vi "Parse Response Message.vi"(6 "Command in":T1, 8 "error in":errorcluster, 11 "Kronos in":refnum<class "Kronos.lvclass">) -> (0 "error out":errorcluster, 3 "Kronos out":refnum<class "Kronos.lvclass">)   [LabVIEW 2018, in "Kronos.lvlib" / "Kronos.lvclass"]
uses:
  Kronos.lvclass
  PPLs/Laser/Parent/Laser.lvlibp/Custom Controls/Command List.ctl
  PPLs/Laser/Parent/Laser.lvlibp/Laser.lvclass
  C:/AME Test Engineering/LabVIEW/PPLs/Laser/Parent/Laser.lvlibp/Laser.lvclass
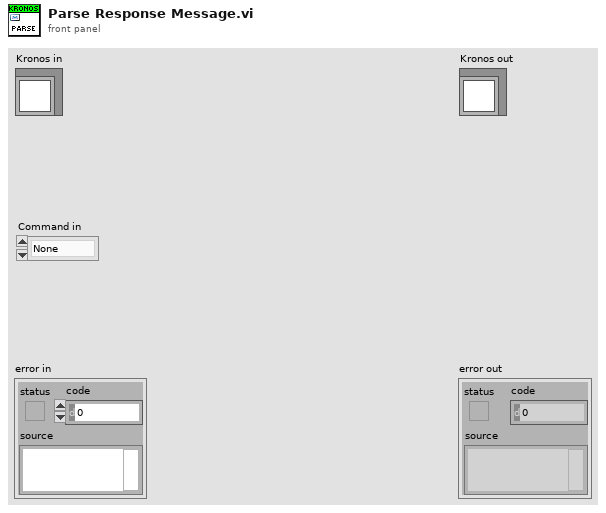
[diagram p1: front panel]
types:
  T1 = typedef "Laser.lvlibp/Laser.lvclass/Command List.ctl" = enum16{"None", "Config?", "Volt?", "ThCase?", "STS?", "Mon?", "Help?", "HB", "Verbose", "Spnt", "Ext", "PRF", "Start", "Stop", "PRF?", "State?", "Status?", "Stat?", "Read HB", "Logon", "Poutmax", "saveconfig", "Reset", "Poutmax?", "PoutCommandMax", "PoutCommandMax?", "FreqMin", "FreqMin?"}
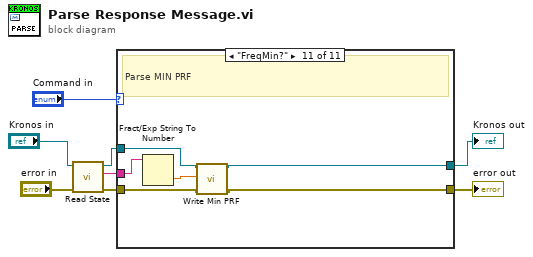
[diagram p0: block diagram]
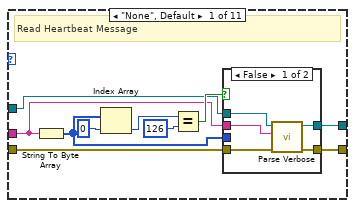
[diagram p2: hidden frame]
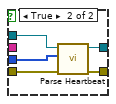
[diagram p3: hidden frame]
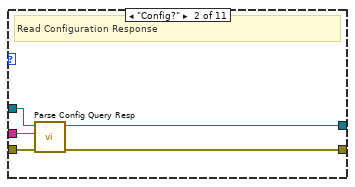
[diagram p4: hidden frame]
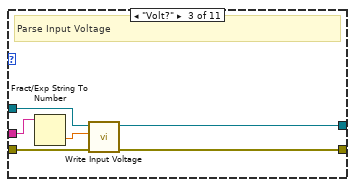
[diagram p5: hidden frame]
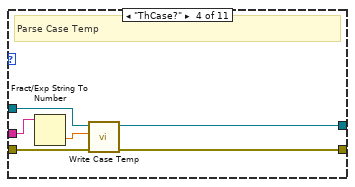
[diagram p6: hidden frame]
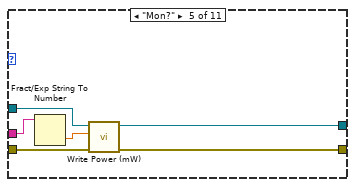
[diagram p7: hidden frame]
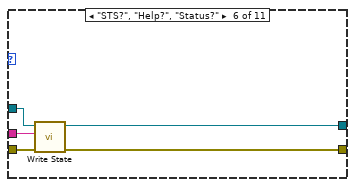
[diagram p8: hidden frame]
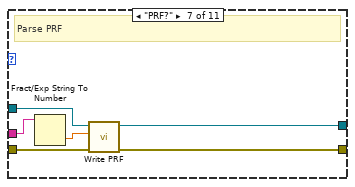
[diagram p9: hidden frame]
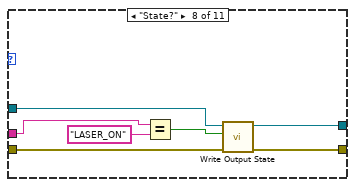
[diagram p10: hidden frame]
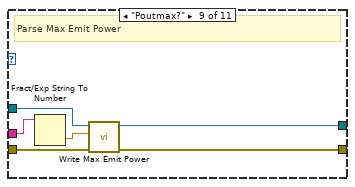
[diagram p11: hidden frame]
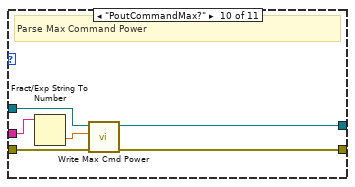
[diagram p12: hidden frame]
diagram:
  n1 = call "Read State.vi"("error in (no error)"="error in", "Laser in"="Kronos in") -> ("error out"=w2:errorcluster, "State"=w6:string, "Laser out"=w5:refnum<class "Kronos.lvclass">)  [unwired: 7 in]
  n2 = case shown="\"FreqMin?\"" "Command in" {
    tunnel: w6 -> [w13 w33 w39 w45 w51 w56 w62 w69 w75 w81 w87]
    tunnel: w5 -> [w12 w32 w37 w43 w49 w55 w60 w66 w73 w79 w86]
    tunnel: [w11 w31 w36 w42 w48 w52 w59 w65 w72 w78 w85] -> w4
    tunnel: [w10 w30 w35 w41 w46 w53 w58 w63 w71 w77 w84] -> w3
    tunnel: w2 -> [w9 w29 w34 w40 w47 w54 w57 w64 w70 w76 w83]
    frame "None", Default {
      # "Read Heartbeat Message"
      n3 = String To Byte Array(string=w13) -> (unsigned byte array=w14:u8[])
      n4 = Index Array(array=w14, index=0) -> (element=w18:u8)
      n5 = Equal?(x=w18, y=u8 126) -> (x = y?=w15:bool)
      n6 = case shown="False" w15 {
        tunnel: w14 -> [_ w28]
        tunnel: w13 -> [w23 _]
        tunnel: w12 -> [w22 w27]
        tunnel: [w21 w26] -> w11
        tunnel: [w19 w25] -> w10
        tunnel: w9 -> [w20 w24]
        frame False {
          n7 = call "Parse Verbose.vi"("error in"=w20, "Heartbeat in"=w23, "Kronos in"=w22) -> ("error out"=w19:errorcluster, "Kronos out"=w21:refnum<class "Kronos.lvclass">)  [unwired: 7 in]
        }
        frame True {
          n8 = call "Parse Heartbeat.vi"("error in"=w24, "Hearbeat in"=w28, "Kronos in"=w27) -> ("error out"=w25:errorcluster, "Kronos out"=w26:refnum<class "Kronos.lvclass">)  [unwired: 7 in]
        }
      }
    }
    frame "Config?" {
      # "Read Configuration Response"
      n9 = call "Parse Config Query Resp.vi"("error in"=w29, "State"=w33, "Kronos in"=w32) -> ("error out"=w30:errorcluster, "Kronos out"=w31:refnum<class "Kronos.lvclass">)  [unwired: 7 in]
    }
    frame "Volt?" {
      # "Parse Input Voltage"
      n10 = Fract/Exp String To Number(string=w39) -> (number=w38:dbl)  [unwired: 3 in, 1 out]
      n11 = call "Write Input Voltage.vi"("error in (no error)"=w34, "Input Voltage"=w38, "Laser in"=w37) -> ("error out"=w35:errorcluster, "Laser out"=w36:refnum<class "Kronos.lvclass">)  [unwired: 7 in]
    }
    frame "ThCase?" {
      # "Parse Case Temp"
      n12 = Fract/Exp String To Number(string=w45) -> (number=w44:dbl)  [unwired: 3 in, 1 out]
      n13 = call "Write Case Temp.vi"("error in (no error)"=w40, "Case Temp"=w44, "Laser in"=w43) -> ("error out"=w41:errorcluster, "Laser out"=w42:refnum<class "Kronos.lvclass">)  [unwired: 7 in]
    }
    frame "Mon?" {
      n14 = Fract/Exp String To Number(string=w51) -> (number=w50:dbl)  [unwired: 3 in, 1 out]
      n15 = call "Write Power (mW).vi"("error in (no error)"=w47, "Power (mW)"=w50, "Laser in"=w49) -> ("error out"=w46:errorcluster, "Laser out"=w48:refnum<class "Kronos.lvclass">)  [unwired: 7 in]
    }
    frame "STS?", "Help?", "Status?" {
      n16 = call "Write State.vi"("error in (no error)"=w54, "State"=w56, "Laser in"=w55) -> ("error out"=w53:errorcluster, "Laser out"=w52:refnum<class "Kronos.lvclass">)  [unwired: 7 in]
    }
    frame "PRF?" {
      # "Parse PRF"
      n17 = Fract/Exp String To Number(string=w62) -> (number=w61:dbl)  [unwired: 3 in, 1 out]
      n18 = call "Write PRF.vi"("error in (no error)"=w57, "PRF"=w61, "Laser in"=w60) -> ("error out"=w58:errorcluster, "Laser out"=w59:refnum<class "Kronos.lvclass">)  [unwired: 7 in]
    }
    frame "State?" {
      n19 = Equal?(x=w69, y="LASER_ON") -> (x = y?=w67:bool)
      n20 = call "Write Output State.vi"("error in (no error)"=w64, "Output State"=w67, "Laser in"=w66) -> ("error out"=w63:errorcluster, "Laser out"=w65:refnum<class "Kronos.lvclass">)  [unwired: 7 in]
    }
    frame "Poutmax?" {
      # "Parse Max Emit Power"
      n21 = Fract/Exp String To Number(string=w75) -> (number=w74:dbl)  [unwired: 3 in, 1 out]
      n22 = call "Write Max Emit Power.vi"("error in (no error)"=w70, "Max Emit Power"=w74, "Laser in"=w73) -> ("error out"=w71:errorcluster, "Laser out"=w72:refnum<class "Kronos.lvclass">)  [unwired: 7 in]
    }
    frame "PoutCommandMax?" {
      # "Parse Max Command Power"
      n23 = Fract/Exp String To Number(string=w81) -> (number=w80:dbl)  [unwired: 3 in, 1 out]
      n24 = call "Write Max Cmd Power.vi"("error in (no error)"=w76, "Max Cmd Power"=w80, "Laser in"=w79) -> ("error out"=w77:errorcluster, "Laser out"=w78:refnum<class "Kronos.lvclass">)  [unwired: 7 in]
    }
    frame "FreqMin?" {
      # "Parse MIN PRF"
      n25 = Fract/Exp String To Number(string=w87) -> (number=w82:dbl)  [unwired: 3 in, 1 out]
      n26 = call "Write Min PRF.vi"("error in (no error)"=w83, "Min PRF"=w82, "Laser in"=w86) -> ("error out"=w84:errorcluster, "Laser out"=w85:refnum<class "Kronos.lvclass">)  [unwired: 7 in]
    }
  }
  "error out" <- w3
  "Kronos out" <- w4
